vi "Manual Mode - Read Configurations.vi"   [LabVIEW 2014, in "Associated Power Technologies 8500 Series.lvlib"]
uses:
  <instrlib>/Associated Power Technologies 8500 Series/Associated Power Technologies 8500 Series.lvlib
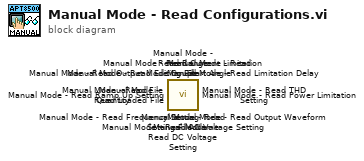
[diagram p0: block diagram]
diagram:
  n1 = call <instrlib>:"Manual Mode - Read Setting File Name.vi"() -> ()  [unwired: 9 in, 3 out]
  n2 = call <instrlib>:"Manual Mode - Read Start Angle.vi"() -> ()  [unwired: 9 in, 3 out]
  n3 = call <instrlib>:"Manual Mode - Read File Quantity.vi"() -> ()  [unwired: 9 in, 3 out]
  n4 = call <instrlib>:"Manual Mode - Read THD Setting.vi"() -> ()  [unwired: 9 in, 3 out]
  n5 = call <instrlib>:"Manual Mode - Read Output Mode Couple.vi"() -> ()  [unwired: 9 in, 3 out]
  n6 = call <instrlib>:"Manual Mode - Read Range.vi"() -> ()  [unwired: 9 in, 3 out]
  n7 = call <instrlib>:"Manual Mode - Read Output Waveform.vi"() -> ()  [unwired: 9 in, 3 out]
  n8 = call <instrlib>:"Manual Mode - Read DC Voltage Setting.vi"() -> ()  [unwired: 9 in, 3 out]
  n9 = call <instrlib>:"Manual Mode - Read Frequency Setting.vi"() -> ()  [unwired: 9 in, 3 out]
  n10 = call <instrlib>:"Manual Mode - Read Ramp Up Setting.vi"() -> ()  [unwired: 9 in, 3 out]
  n11 = call <instrlib>:"Manual Mode - Read Power Limitation.vi"() -> ()  [unwired: 9 in, 3 out]
  n12 = call <instrlib>:"Manual Mode - Read Limitation Delay.vi"() -> ()  [unwired: 9 in, 3 out]
  n13 = call <instrlib>:"Manual Mode - Read Current Limitation.vi"() -> ()  [unwired: 9 in, 3 out]
  n14 = call <instrlib>:"Manual Mode - Read AC Voltage Setting.vi"() -> ()  [unwired: 9 in, 3 out]
  n15 = call <instrlib>:"Manual Mode - Read Editing File.vi"() -> ()  [unwired: 9 in, 3 out]
  n16 = call <instrlib>:"Manual Mode - Read Loaded File.vi"() -> ()  [unwired: 9 in, 3 out]
